vi "GFITS_getKeyvalueFromRemoteDBS.vi"(0 "key name in header":string, 1 "Database RefNum in":T1, 5 "varname":string, 7 "comment":string, 9 "extension":i16=1, 11 "error in (no error)":errorcluster) -> (6 "table out":string[][](table), 10 "datatype":u16=16, 14 "function to use":string, 15 "error out":errorcluster)   [LabVIEW 2016]
uses:
  GFITS_datatypesctl.ctl
  DBSHAND/private/vis/DatabaseHand_RefNum.ctl
  DBSHAND/private/vis/DatabaseHand_Element_Get(string).vi
  DBSHAND/private/vis/DatabaseHand_Element_Get(I32).vi
panel:
  out "remote port":i32=1300
  out "ip address":string="localhost"
  in  "Types":T2={"TBIT"=1, "TBYTE"=11, "TSTRING"=16, "TSHORT"=21, "TLONG"=41, "TFLOAT"=42, "TDOUBLE"=82, "TCOMPLEX"=83, "TDBLCOMPLEX"=163, "TUINT"=30, "TUSHORT"=20, "TULONG"=40, "TINT"=31, "TSBYTE"=12, "TLONGLONG"=81, "TLOGICAL"=14}
  in  "Supported DataTypes":i32(listbox)
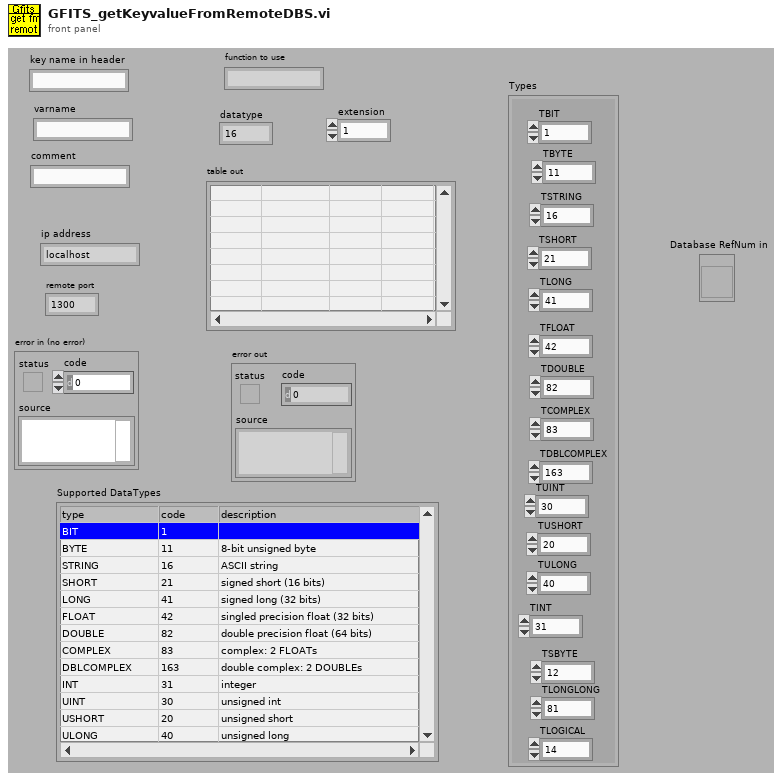
[diagram p1: front panel]
types:
  T1 = typedef "DatabaseHand_RefNum.ctl" = refnum<vi>
  T2 = typedef "GFITS_datatypesctl.ctl" = cluster{"TBIT":i32, "TBYTE":i32, "TSTRING":i32, "TSHORT":i32, "TLONG":i32, "TFLOAT":i32, "TDOUBLE":i32, "TCOMPLEX":i32, "TDBLCOMPLEX":i32, "TUINT":i32, "TUSHORT":i32, "TULONG":i32, "TINT":i32, "TSBYTE":i32, "TLONGLONG":i32, "TLOGICAL":i32}
  T3 = enum16{"Standard", "Buffered", "CRLF", "Immediate"}
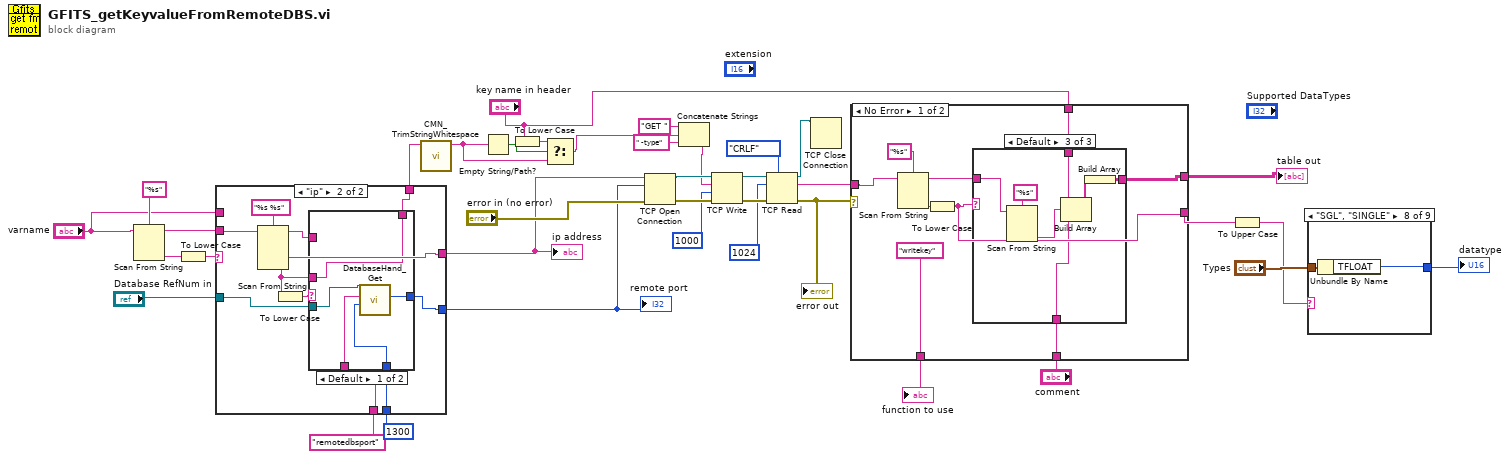
[diagram p0: block diagram]
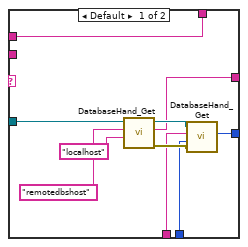
[diagram p2: hidden frame]
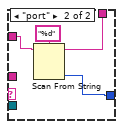
[diagram p3: hidden frame]
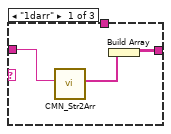
[diagram p4: hidden frame]
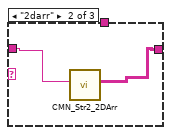
[diagram p5: hidden frame]
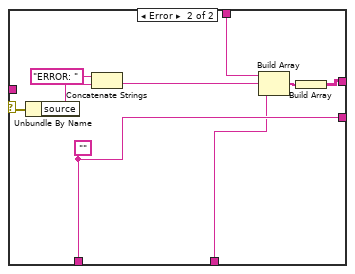
[diagram p6: hidden frame]
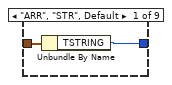
[diagram p7: hidden frame]
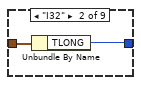
[diagram p8: hidden frame]
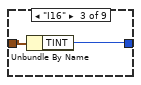
[diagram p9: hidden frame]
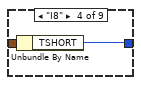
[diagram p10: hidden frame]
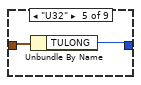
[diagram p11: hidden frame]
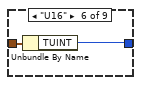
[diagram p12: hidden frame]
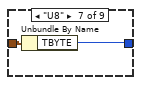
[diagram p13: hidden frame]
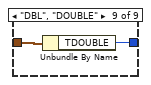
[diagram p14: hidden frame]
diagram:
  n1 = Scan From String(format string="%s", input string="varname") -> (remaining string=w11:string, output 1=w8:string)  [unwired: 2 in, 3 out]
  n2 = To Lower Case(string=w8) -> (all lower case string=w1:string)
  n3 = case shown="\"ip\"" w1 {
    tunnel: w11 -> [_ w58]
    tunnel: "varname" -> [w43 _]
    tunnel: [w43 w50] -> w4
    tunnel: [w42 w56] -> w10
    tunnel: [w41 w52] -> w9
    tunnel: "Database RefNum in" -> [w40 w55]
    tunnel: "remotedbsport" ("name") -> [w39 w54]
    tunnel: 1300 -> [w38 w53]
    frame Default {
      n4 = call-poly "DatabaseHand_Get.vi"("default value"="localhost", "name"="remotedbshost", "Database RefNum in"=w40) -> ("error out"=w46:errorcluster, "value"=w42:string, "Database RefNum out"=w47:T1)  [unwired: 2 in, 4 out]
      n5 = call-poly "DatabaseHand_Get.vi"("error in (no error)"=w46, "default value"=w38, "name"=w39, "Database RefNum in"=w47) -> ("value"=w41:i32)  [unwired: 1 in, 6 out]
    }
    frame "ip" {
      n6 = Scan From String(format string="%s %s", input string=w58) -> (remaining string=w51:string, output 1=w56:string, output 2=w48:string)  [unwired: 2 in, 4 out]
      n7 = To Lower Case(string=w48) -> (all lower case string=w49:string)
      n8 = case shown="Default" w49 {
        tunnel: w55 -> [w63 _]
        tunnel: w54 -> [w62 _]
        tunnel: w53 -> [w61 _]
        tunnel: [w60 w65] -> w52
        tunnel: w51 -> [_ w67]
        tunnel: [w59 w64] -> w50
        tunnel: w48 -> [w59 _]
        frame Default {
          n9 = call-poly "DatabaseHand_Get.vi"("default value"=w61, "name"=w62, "Database RefNum in"=w63) -> ("value"=w60:i32)  [unwired: 2 in, 6 out]
        }
        frame "port" {
          n10 = Scan From String(format string="%d", input string=w67) -> (remaining string=w64:string, output 1=w65:i32)  [unwired: 2 in, 3 out]
        }
      }
    }
  }
  "ip address" <- w10
  "remote port" <- w9
  n11 = call "CMN_TrimStringWhitespace.vi"("string"=w4) -> ("trimmed string"=w3:string)  [unwired: 1 in, 8 out]
  n12 = Empty String/Path?(string/path=w3) -> (empty?=w28:bool)
  n13 = To Lower Case(string="key name in header") -> (all lower case string=w29:string)
  n14 = Select(t=w29, s=w28, f=w3) -> (s? t:f=w27:string)
  n15 = TCP Open Connection(address=w10, remote port or service name=w9, error in (no error)="error in (no error)") -> (connection ID=w35:refnum<k5>, error out=w34:errorcluster)  [unwired: 2 out]
  n16 = Concatenate Strings("GET " ("string"), w27, " -type" ("string")) -> (w32:string)
  n17 = TCP Write(connection ID=w35, data in=w32, error in (no error)=w34, 9:1000 ("timeout ms (25000)")) -> (connection ID out=w30:refnum<k5>, error out=w31:errorcluster)  [unwired: 1 out]
  n18 = TCP Read(connection ID=w30, bytes to read=1024, error in (no error)=w31, 7:T3."CRLF" ("mode (standard)")) -> (connection ID out=w25:refnum<k5>, data out=w24:string, error out=w21:errorcluster)  [unwired: 1 out]
  "error out" <- w21
  n19 = TCP Close Connection(connection ID=w25) -> ()  [unwired: 1 in, 3 out]
  n20 = case shown="No Error" w21 {
    selector: w21 -> [_ w97]
    tunnel: w24 -> [w76 _]
    tunnel: [w70 w94] -> w23
    tunnel: ["writekey" w94] -> w20
    tunnel: "key name in header" -> [w72 w92]
    tunnel: [w69 w89] -> w17
    tunnel: "comment" -> [w68 w91]
    frame No Error {
      n21 = Scan From String(format string="%s", input string=w76) -> (remaining string=w71:string, output 1=w73:string)  [unwired: 2 in, 3 out]
      n22 = To Lower Case(string=w73) -> (all lower case string=w70:string)
      n23 = case shown="Default" w70 {
        tunnel: w72 -> [_ _ w88]
        tunnel: w71 -> [w79 w81 w87]
        tunnel: [w77 w80 w83] -> w69
        tunnel: w68 -> [_ _ w82]
        frame "1darr" {
          n24 = call "CMN_Str2Arr.vi"("string in"=w79) -> ("Array out"=w78:string[])  [unwired: 3 in, 7 out]
          n25 = Build Array(w78) -> (w77:string[][])
        }
        frame "2darr" {
          n26 = call "CMN_Str2_2DArr.vi"("multi line string in"=w81) -> ("array out"=w80:string[][])  [unwired: 1 in, 9 out]
        }
        frame Default {
          n27 = Scan From String(format string="%s", input string=w87) -> (output 1=w85:string)  [unwired: 2 in, 4 out]
          n28 = Build Array(w88, w85, w82) -> (w84:string[])
          n29 = Build Array(w84) -> (w83:string[][])
        }
      }
    }
    frame Error {
      w94 = ""
      n30 = Unbundle By Name(w97) -> ("source"=w96:string)
      n31 = Concatenate Strings("ERROR: " ("string"), w96) -> (w93:string)
      n32 = Build Array(w92, w93, w91) -> (w90:string[])
      n33 = Build Array(w90) -> (w89:string[][])
    }
  }
  "function to use" <- w20
  "table out" <- w17
  n34 = To Upper Case(1:w23) -> (0:w13:string)
  n35 = case shown="\"SGL\", \"SINGLE\"" w13 {
    tunnel: [w99 w101 w103 w105 w107 w109 w111 w113 w115] -> w36
    tunnel: "Types" -> [w98 w100 w102 w104 w106 w108 w110 w112 w114]
    frame "ARR", "STR", Default {
      n36 = Unbundle By Name(w98) -> ("TSTRING"=w99:i32)
    }
    frame "I32" {
      n37 = Unbundle By Name(w100) -> ("TLONG"=w101:i32)
    }
    frame "I16" {
      n38 = Unbundle By Name(w102) -> ("TINT"=w103:i32)
    }
    frame "I8" {
      n39 = Unbundle By Name(w104) -> ("TSHORT"=w105:i32)
    }
    frame "U32" {
      n40 = Unbundle By Name(w106) -> ("TULONG"=w107:i32)
    }
    frame "U16" {
      n41 = Unbundle By Name(w108) -> ("TUINT"=w109:i32)
    }
    frame "U8" {
      n42 = Unbundle By Name(w110) -> ("TBYTE"=w111:i32)
    }
    frame "SGL", "SINGLE" {
      n43 = Unbundle By Name(w112) -> ("TFLOAT"=w113:i32)
    }
    frame "DBL", "DOUBLE" {
      n44 = Unbundle By Name(w114) -> ("TDOUBLE"=w115:i32)
    }
  }
  "datatype" <- w36
